vi "set_camera_attributes.vi"(0 "Session In":T1, 1 "Brightness":dbl, 2 "Gain":dbl, 3 "Shutter":dbl, 4 "error in (no error)":errorcluster) -> (5 "Session Out":T1, 6 "error out":errorcluster)   [LabVIEW 2017]
uses:
  <vilib>/userdefined/High Color/IMAQdx.ctl
  <resource>/objmgr/imaqdx.rc
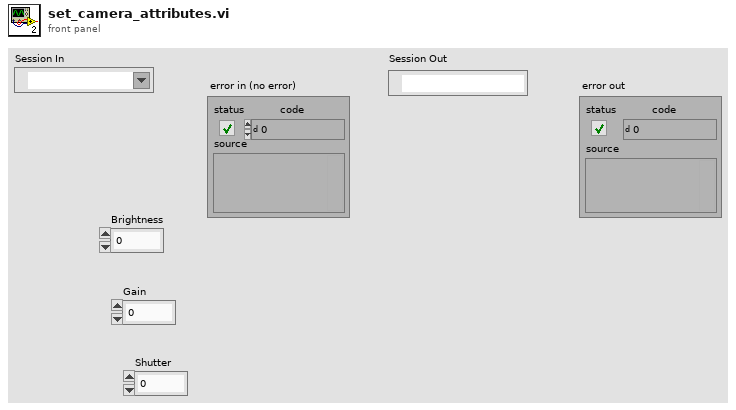
[diagram p1: front panel]
types:
  T1 = typedef "IMAQdx.ctl" = refnum<k21>
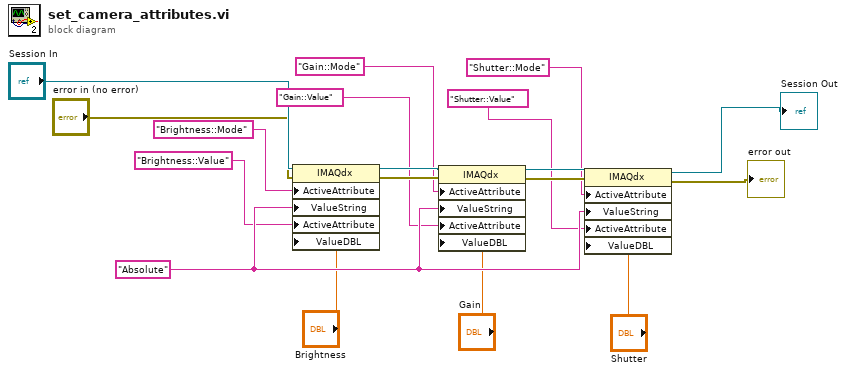
[diagram p0: block diagram]
diagram:
  w14 = "Absolute"
  n1 = property class="IMAQdx"(reference="Session In", error in="error in (no error)", "ActiveAttribute"="Brightness::Mode", "ValueString"=w14, "ActiveAttribute"="Brightness::Value", "ValueDBL"="Brightness") -> (reference out=w18:T1, error out=w16:errorcluster)
  n2 = property class="IMAQdx"(reference=w18, error in=w16, "ActiveAttribute"="Gain::Mode", "ValueString"=w14, "ActiveAttribute"="Gain::Value", "ValueDBL"="Gain") -> (reference out=w17:T1, error out=w15:errorcluster)
  n3 = property class="IMAQdx"(reference=w17, error in=w15, "ActiveAttribute"="Shutter::Mode", "ValueString"=w14, "ActiveAttribute"="Shutter::Value", "ValueDBL"="Shutter") -> (reference out=→"Session Out":T1, error out=→"error out":errorcluster)
